vi "Switch Channels.vi"   [LabVIEW 2020, in "Keithley 27XX.lvlib"]
doc: "This VI closes/opens channels on installed switching cards. This is automatically handled when using a scan list to take measurements."
uses:
  <instrlib>/Keithley 27XX/Keithley 27XX.lvlib
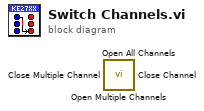
[diagram p0: block diagram]
diagram:
  n1 = call <instrlib>:"Open Multiple Channels.vi"() -> ()  [unwired: 14 in, 2 out]
  n2 = call <instrlib>:"Open All Channels.vi"() -> ()  [unwired: 14 in, 2 out]
  n3 = call <instrlib>:"Close Multiple Channel.vi"() -> ()  [unwired: 14 in, 2 out]
  n4 = call <instrlib>:"Close Channel.vi"() -> ()  [unwired: 14 in, 2 out]
